vi "init.vi"(4 "Measurements":string, 6 "SA Frequency (Hz)":dbl=0.0001 format="%.3p", 7 "Prepend Result Name":bool, 8 "error in (no error)":errorcluster, 9 "Number of Slots":i32=1, 10 "Measurement Name":string, 11 "SA Pin":string) -> (0 "error out":errorcluster, 3 "Skyworks_PA_Modeswitch_out":refnum<class "HiSi_SpecAn_IQSLOT.lvclass">)   [LabVIEW 2018, in "SeqAuto Evaluations.lvlib" / "HiSi_SpecAn_IQSLOT.lvclass"]
uses:
  HiSi_SpecAn_IQSLOT.lvclass
  C:/Sequence Automation/Plugins/SeqAuto IEvaluation.lvlibp/SeqAuto IEvaluation.lvclass
  HiSi_SpecAn_IQSLOT.lvclass/HiSi_SpecAn_IQSLOT.ctl
  Plugins/SeqAuto IEvaluation.lvlibp/Write Measurement Name.vi
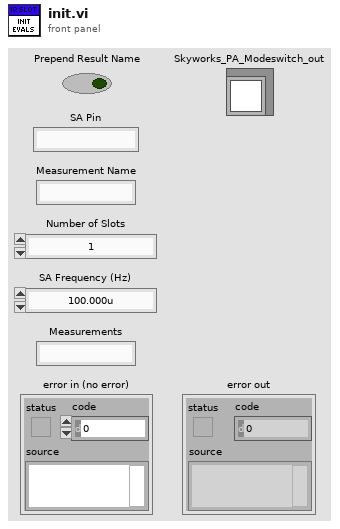
[diagram p1: front panel]
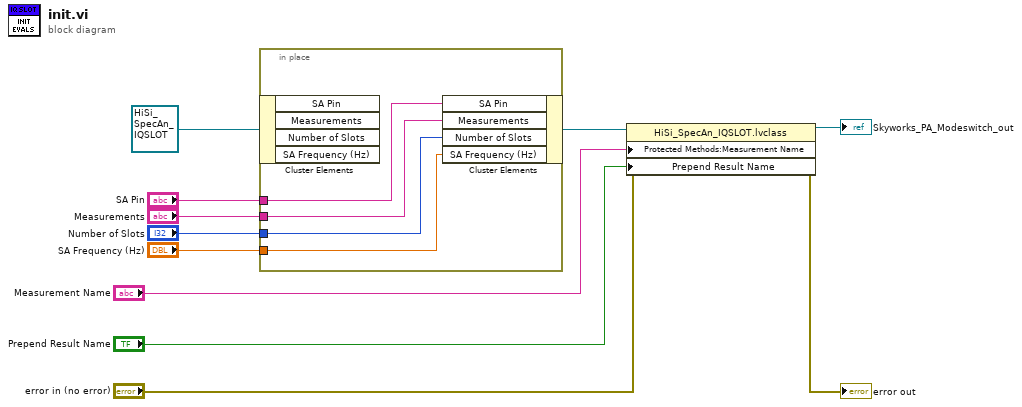
[diagram p0: block diagram]
diagram:
  n1 = in-place {
    in-place-border: "SA Pin" -> [w15]
    in-place-border: "Measurements" -> [w14]
    in-place-border: "Number of Slots" -> [w13]
    in-place-border: "SA Frequency (Hz)" -> [w12]
    n2 = in-place-cluster #1(refnum<class "HiSi_SpecAn_IQSLOT.lvclass"> refnum ("Skyworks_2G_PVT in")) -> ()  [unwired: 4 out]
    n3 = in-place-cluster #1("SA Pin"=w15, "Measurements"=w14, "Number of Slots"=w13, "SA Frequency (Hz)"=w12) -> (w3:refnum<class "HiSi_SpecAn_IQSLOT.lvclass">)
  }
  n4 = property class="HiSi_SpecAn_IQSLOT.lvclass"(reference=w3, error in="error in (no error)", "Protected Methods:Measurement Name"="Measurement Name", "Prepend Result Name"="Prepend Result Name") -> (reference out=→"Skyworks_PA_Modeswitch_out":refnum<class "HiSi_SpecAn_IQSLOT.lvclass">, error out=→"error out":errorcluster)
